vi "HX711.vi"() -> ()   [LabVIEW 2019]
uses:
  Data.ctl
  State.ctl
  <vilib>/rvi/Emulation/niFpgaSctlEmulationGetInTimedLoop.vi
  <vilib>/rvi/Emulation/niFpgaProcessEmulError.vi
  <vilib>/rvi/Emulation/niFpgaGetClockAttributes.vi
  <vilib>/rvi/Emulation/niFpgaEmulationReportErrorSimple.vi
  <vilib>/rvi/eio/common/nirviEmuTemplateMethod_errors.vi
  <vilib>/rvi/Emulation/niFpgaCriticalErrorInLSC.vi
  <vilib>/eio/EIONode/EIONode.xnode
panel:
  out "Data array":i32[](array[numeric])
  in  "stop":bool
  in  "Gain/ChannelSelect":T1(ring)
  in  "PowerDown?":bool
  out "Data":i32
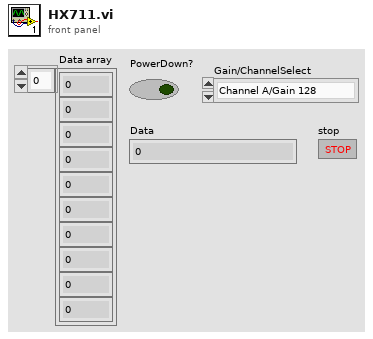
[diagram p1: front panel]
types:
  T1 = enum16{"Channel A/Gain 128", "Channel A/Gain 64", "Channel B/Gain 32"}
  T2 = typedef "State.ctl" = enum16{"PowerUp", "PowerDown", "Gain/ChannelSelect", "ReadData", "ClockLow", "ClockHigh", "ConvertData", "RetrievalReady?"}
  T3 = typedef "Data.ctl" = cluster{"DT":bool, "SCK":bool, "2's Data":i32, "PulseCount":u8, "DelayTime":u8, "Data":i32, "PowerDown?":bool, "Gain/ChannelSelect":enum16{"Channel A/Gain 128", "Channel A/Gain 64", "Channel B/Gain 32"}}
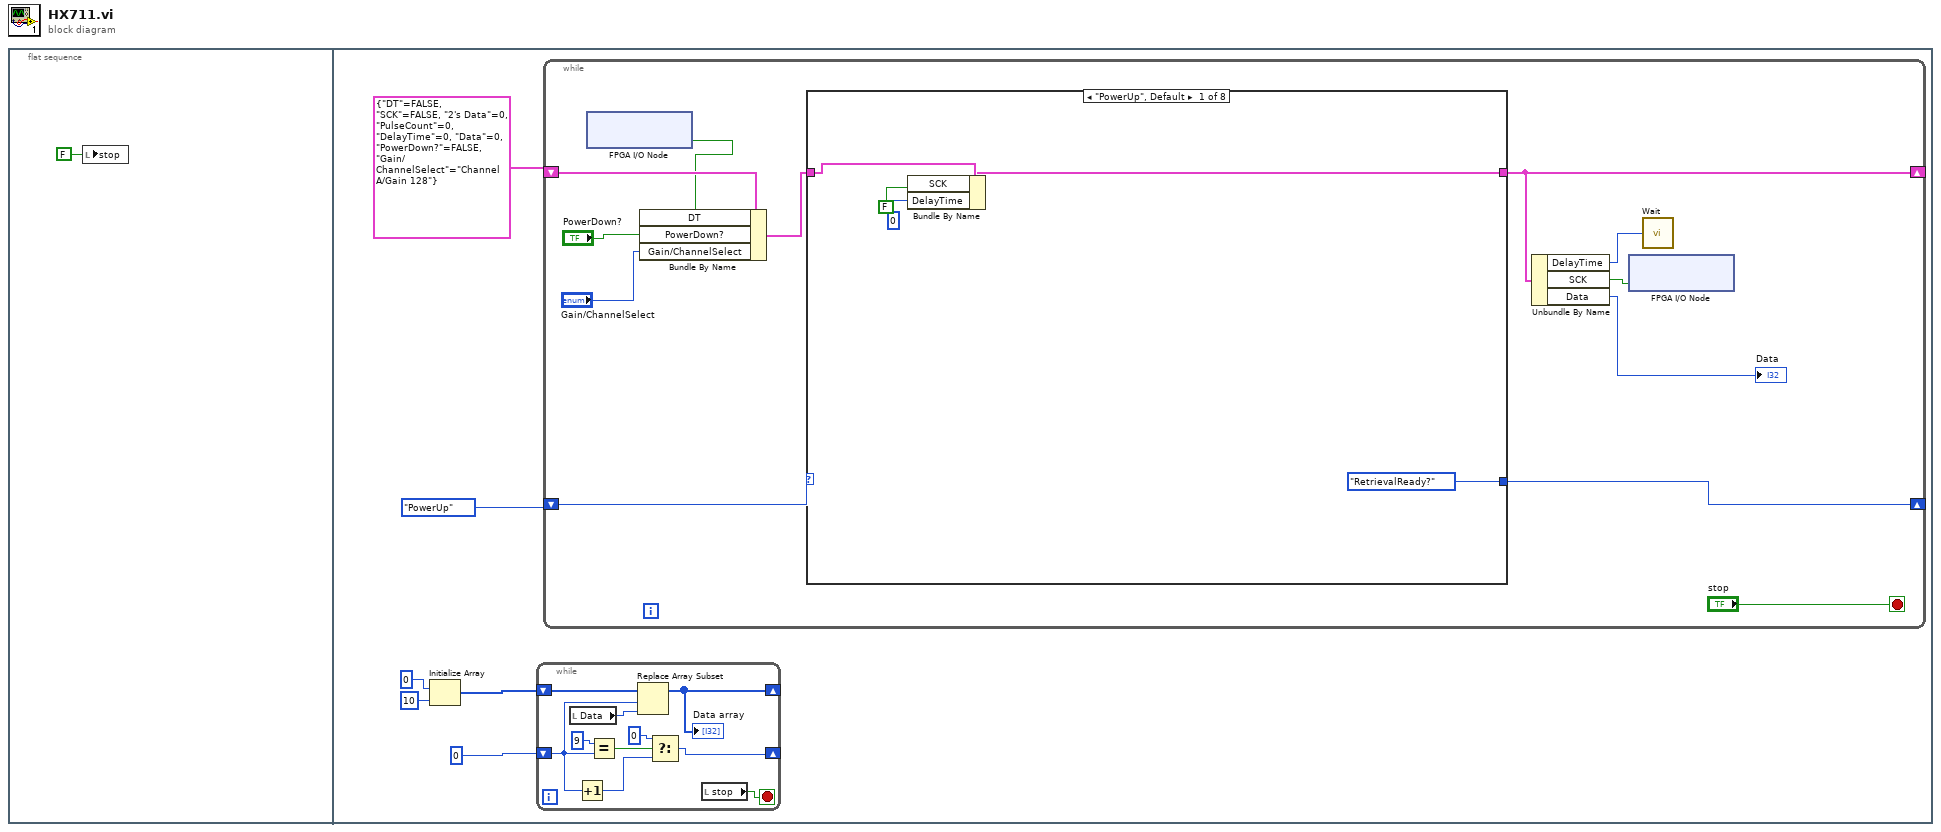
[diagram p0: block diagram]
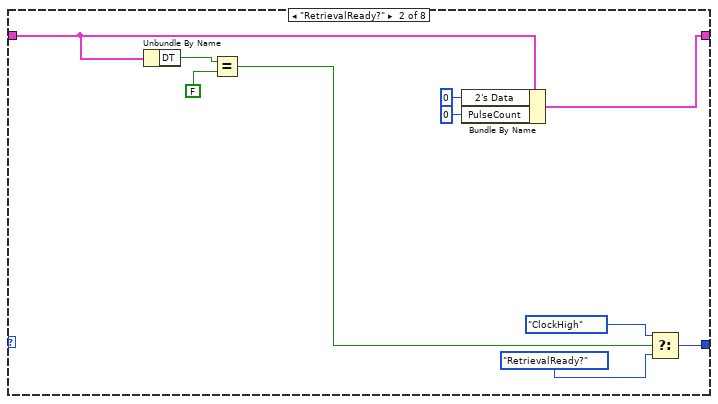
[diagram p2: hidden frame]
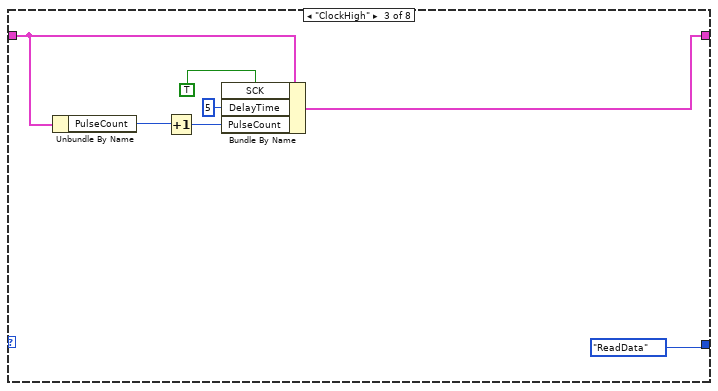
[diagram p3: hidden frame]
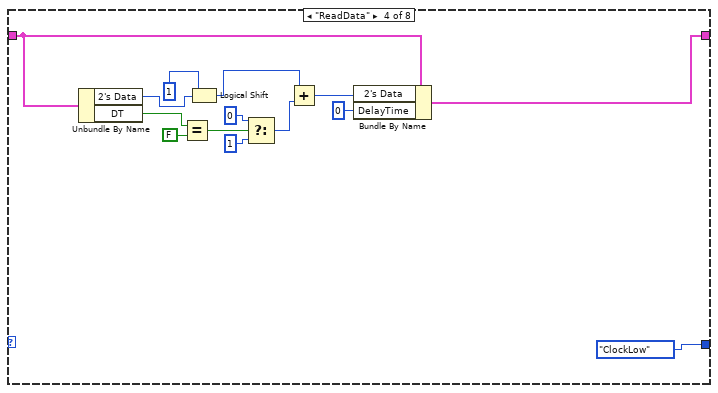
[diagram p4: hidden frame]
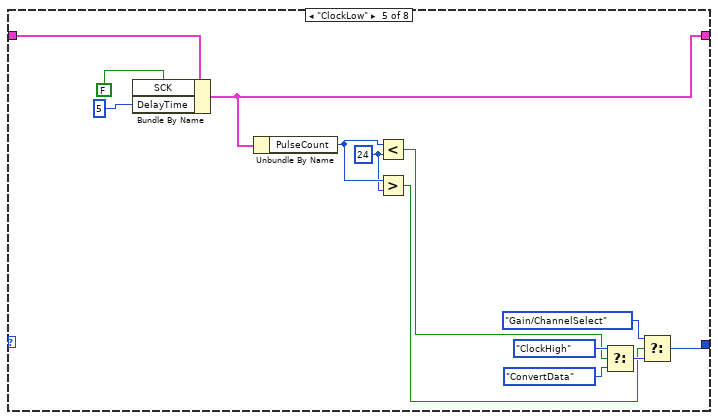
[diagram p5: hidden frame]
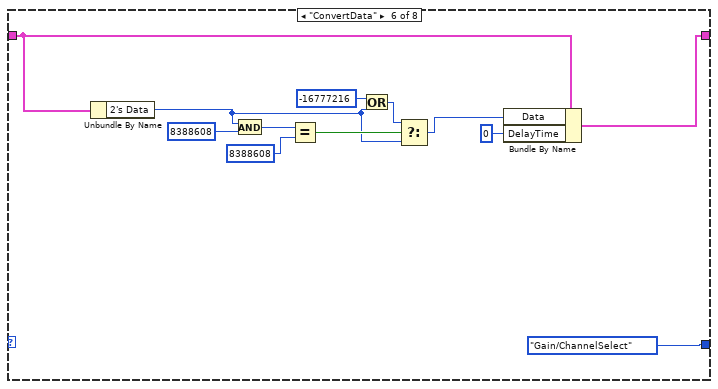
[diagram p6: hidden frame]
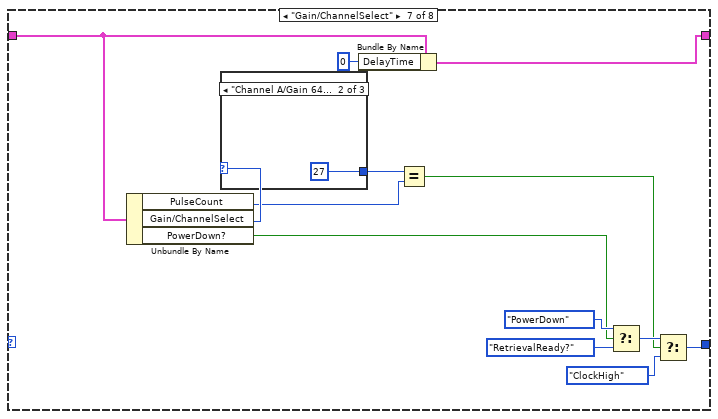
[diagram p7: hidden frame]
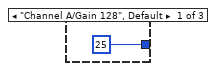
[diagram p8: hidden frame]
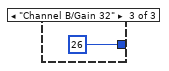
[diagram p9: hidden frame]
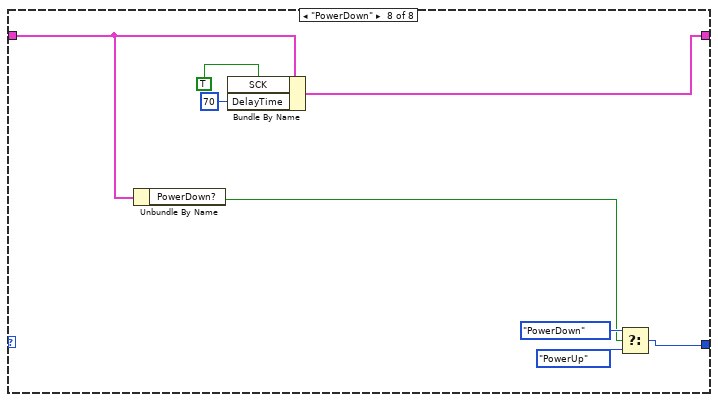
[diagram p10: hidden frame]
diagram:
  n1 = flat-sequence {
    frame #0 {
      n2 = local write "stop"(FALSE) -> ()
    }
    frame #1 {
      n3 = Initialize Array(0 ("Data"), 10 ("dimension size")) -> (w7:i32[])
      n4 = while {
        shift-right: [w9] -> _
        shift-left: w7 -> [w10]
        shift-right: [w15] -> _
        shift-left: 0 ("index") -> [w11]
        stop <- w8 stop-if-true
        n5 = local read "Data"() -> (w17:i32)
        n6 = Increment(x=w11) -> (x+1=w14:i32)
        n7 = Equal?(x=9, y=w11) -> (x = y?=w12:bool)
        n8 = Replace Array Subset(array=w10, new element=w17, index=w11) -> (w9:i32[])
        "Data array" <- w9
        n9 = Select(t=0 ("index"), s=w12, f=w14) -> (s? t:f=w15:i32)
        n10 = local read "stop"() -> (w8:bool)
      }
      n11 = while {
        shift-right: [w20] -> _
        shift-left: T3 {"DT"=FALSE, "SCK"=FALSE, "2's Data"=0, "PulseCount"=0, "DelayTime"=0, "Data"=0, "PowerDown?"=FALSE, "Gain/ChannelSelect"=enum."Channel A/Gain 128"} ("Data") -> [w26]
        shift-right: [w27] -> _
        shift-left: State."PowerUp" ("State") -> [w29]
        stop <- "stop" stop-if-true
        n12 = xnode "FPGA I/O Node"() -> ("Mod8/DIO0"=w24:bool)  [unwired: 1 in, 1 out]
        n13 = Bundle By Name(cluster=w26, "DT"=w24, "PowerDown?"="PowerDown?", "Gain/ChannelSelect"="Gain/ChannelSelect") -> (w25:T3)
        n14 = case shown="\"PowerUp\", Default" w29 {
          tunnel: w25 -> [w34 w38 w47 w52 w78 w83 w93 w108]
          tunnel: [w32 w37 w51 w54 w73 w82 w92 w114] -> w20
          tunnel: [State."RetrievalReady?" ("State") w40 State."ReadData" ("State") State."ClockLow" ("State") w74 State."Gain/ChannelSelect" ("State") w100 w109] -> w27
          frame "PowerUp", Default {
            n15 = Bundle By Name(cluster=w34, "SCK"=FALSE, "DelayTime"=u8 0) -> (w32:T3)
          }
          frame "RetrievalReady?" {
            n16 = Unbundle By Name(w38) -> ("DT"=w44:bool)
            n17 = Equal?(x=w44, y=FALSE) -> (x = y?=w39:bool)
            n18 = Bundle By Name(cluster=w38, "2's Data"=0, "PulseCount"=u8 0) -> (w37:T3)
            n19 = Select(t=State."ClockHigh" ("State"), s=w39, f=State."RetrievalReady?" ("State")) -> (s? t:f=w40:T2)
          }
          frame "ClockHigh" {
            n20 = Unbundle By Name(w47) -> ("PulseCount"=w46:u8)
            n21 = Increment(x=w46) -> (x+1=w45:u8)
            n22 = Bundle By Name(cluster=w47, "SCK"=TRUE, "DelayTime"=u8 5, "PulseCount"=w45) -> (w51:T3)
          }
          frame "ReadData" {
            n23 = Unbundle By Name(w52) -> ("2's Data"=w65:i32, "DT"=w63:bool)
            n24 = Equal?(x=w63, y=FALSE ("SCK")) -> (x = y?=w61:bool)
            n25 = Logical Shift(y=i16 1, x=w65) -> (x << y=w60:i32)
            n26 = Select(t=0 ("DelayTime"), s=w61, f=1 ("DelayTime")) -> (s? t:f=w57:i32)
            n27 = Add(x=w60, y=w57) -> (x+y=w56:i32)
            n28 = Bundle By Name(cluster=w52, "2's Data"=w56, "DelayTime"=u8 0) -> (w54:T3)
          }
          frame "ClockLow" {
            w67 = u8 24 ("y")
            n29 = Bundle By Name(cluster=w78, "SCK"=FALSE, "DelayTime"=u8 5) -> (w73:T3)
            n30 = Unbundle By Name(w73) -> ("PulseCount"=w68:u8)
            n31 = Less?(x=w68, y=w67) -> (x < y?=w70:bool)
            n32 = Greater?(x=w68, y=w67) -> (0:w66:bool)
            n33 = Select(t=State."ClockHigh" ("State"), s=w70, f=State."ConvertData" ("State")) -> (s? t:f=w69:T2)
            n34 = Select(t=State."Gain/ChannelSelect" ("State"), s=w66, f=w69) -> (s? t:f=w74:T2)
          }
          frame "ConvertData" {
            n35 = Unbundle By Name(w83) -> ("2's Data"=w84:i32)
            n36 = And(x=w84, y=8388608) -> (x .and. y?=w89:i32)
            n37 = Equal?(x=w89, y=8388608) -> (x = y?=w87:bool)
            n38 = Or(x=-16777216 ("y"), y=w84) -> (x .or. y?=w85:i32)
            n39 = Select(t=w85, s=w87, f=w84) -> (s? t:f=w80:i32)
            n40 = Bundle By Name(cluster=w83, "Data"=w80, "DelayTime"=u8 0) -> (w82:T3)
          }
          frame "Gain/ChannelSelect" {
            n41 = Unbundle By Name(w93) -> ("PulseCount"=w96:u8, "Gain/ChannelSelect"=w98:T1, "PowerDown?"=w99:bool)
            n42 = case shown="\"Channel A/Gain 64\"" w98 {
              tunnel: [u8 25 ("PulseCount") u8 27 ("PulseCount") u8 26 ("PulseCount")] -> w97
              frame "Channel A/Gain 128", Default {
              }
              frame "Channel A/Gain 64" {
              }
              frame "Channel B/Gain 32" {
              }
            }
            n43 = Bundle By Name(cluster=w93, "DelayTime"=u8 0) -> (w92:T3)
            n44 = Equal?(x=w97, y=w96) -> (x = y?=w94:bool)
            n45 = Select(t=State."PowerDown" ("State"), s=w99, f=State."RetrievalReady?" ("State")) -> (s? t:f=w95:T2)
            n46 = Select(t=w95, s=w94, f=State."ClockHigh" ("State")) -> (s? t:f=w100:T2)
          }
          frame "PowerDown" {
            n47 = Unbundle By Name(w108) -> ("PowerDown?"=w107:bool)
            n48 = Bundle By Name(cluster=w108, "SCK"=TRUE, "DelayTime"=u8 70) -> (w114:T3)
            n49 = Select(t=State."PowerDown" ("State"), s=w107, f=State."PowerUp" ("State")) -> (s? t:f=w109:T2)
          }
        }
        n50 = Unbundle By Name(w20) -> ("DelayTime"=w28:u8, "SCK"=w19:bool, "Data"=→"Data":i32)
        n51 = xnode "FPGA I/O Node"("Mod8/DIO1"=w19) -> ()  [unwired: 1 in, 1 out]
        n52 = call "Wait"("Count(uSec)"=w28) -> ()  [unwired: 1 out]
      }
    }
  }
